vi "_XNET UDP Socket Multicast Open SubVI.vi"(5 "mode":u32(ring)=2 items=["Write Only"=1, "Read Only"=2, "Read Write"=3], 6 "local interface":string, 7 "stack":refnum<k21>, 8 "error in":errorcluster, 9 "time-to-live":u8=1, 10 "multicast address":string, 11 "local port":u16) -> (0 "error out":errorcluster, 2 "actual local port":u16, 3 "socket":refnum<k20>)   [LabVIEW 2018]
doc: "Opens a UDP multicast socket to send a single datagram to multiple receivers in parallel on the port you specify."
uses:
  nixlvapi.dll
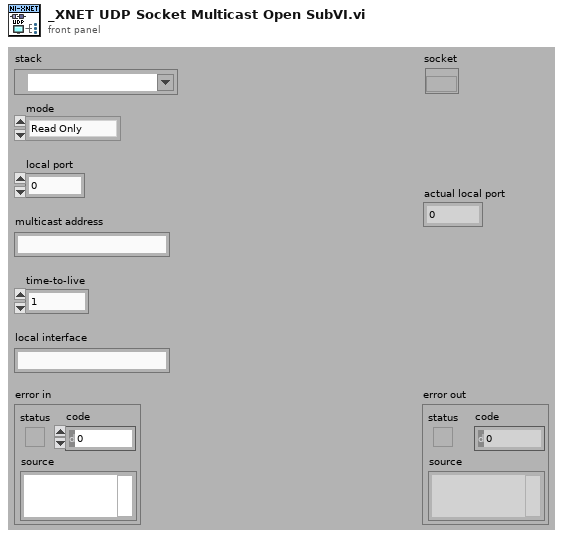
[diagram p1: front panel]
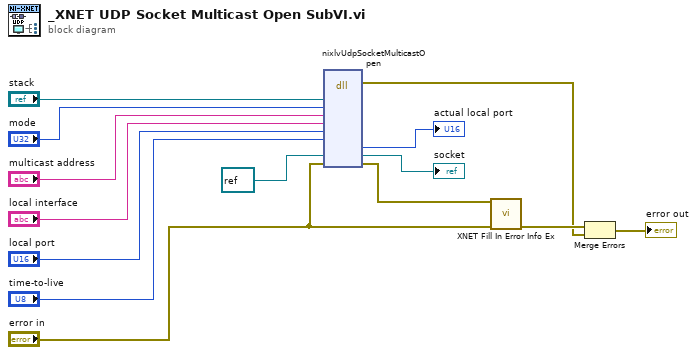
[diagram p0: block diagram]
diagram:
  n1 = dll-call lib="nixlvapi.*" fn="nixlvUdpSocketMulticastOpen" label="Call Library"("stackRef"="stack", "mode"="mode", "multicastAddress"="multicast address", "localInterface"="local interface", "localPort"="local port", "timeToLive"="time-to-live", "socketRefObjPtr"=refnum<k20> refnum ("socket"), "errorInOut"="error in") -> (error out=w12:errorcluster, "actualLocalPort"=→"actual local port":u16, "socketRefObjPtr"=→"socket":refnum<k20>, "errorInOut"=w14:errorcluster)  [unwired: 3 in, 9 out]
  n2 = call "XNET Fill In Error Info Ex.vi"("error xnet"=w14, "error in"="error in") -> ("error out"=w13:errorcluster)  [unwired: 13 in]
  n3 = Merge Errors(w13, w12) -> (→"error out":errorcluster)
